vi "Kalp Atış Hızı Monitörü.vi"() -> ()   [LabVIEW 2017]
uses:
  <vilib>/LabVIEW Interface for Arduino/Type Defs/Digital Pin.ctl
  <vilib>/LabVIEW Interface for Arduino/Type Defs/Pin Mode.ctl
  <vilib>/LabVIEW Interface for Arduino/LabVIEW Interface for Arduino.lvlib
  <vilib>/ptbypt/NI_PtbyPt.lvlib
panel:
  out "Waveform Chart":u8(graph)
  out "Kalp Atımı":bool
  out "Kalp Atış Sayısı":i32
  in  "Çıkış":bool
  in  "Digital Pin":T1
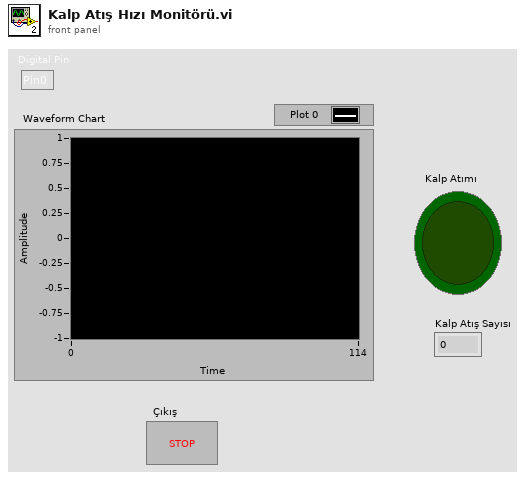
[diagram p1: front panel]
types:
  T1 = typedef "LabVIEW Interface for Arduino.lvlib/Digital Pin.ctl" = enum8{"Pin0", "Pin1", "Pin2", "Pin3", "Pin4", "Pin5", "Pin6", "Pin7", "Pin8", "Pin9", "Pin10", "Pin11", "Pin12", "Pin13"}
  T2 = typedef "LabVIEW Interface for Arduino.lvlib/Arduino Resource.ctl" = cluster{"VISA resource":refnum<visa-resource-name>, "Board Type":T3, "Connection Type":enum8{"USB / Serial"}, "Bytes Per Packet (15)":u8}
  T3 = typedef "LabVIEW Interface for Arduino.lvlib/Board Type.ctl" = enum16{"Uno", "Dimuelanove w/Atmega 328", "Mega 2560"}
  T4 = typedef "LabVIEW Interface for Arduino.lvlib/Pin Mode.ctl" = enum8{"Input", "Output"}
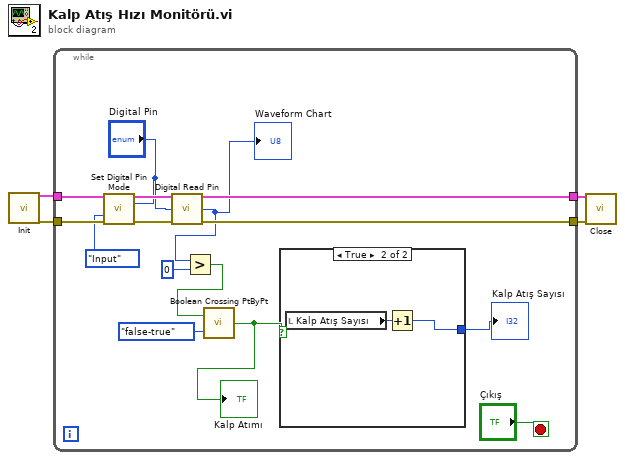
[diagram p0: block diagram]
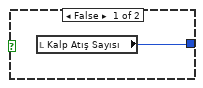
[diagram p2: hidden frame]
diagram:
  n1 = call <vilib>:"Init.vi"() -> ("Arduino Resource"=w2:T2, "error out"=w1:errorcluster)  [unwired: 18 in]
  n2 = while {
    tunnel: w2 -> [w15]
    tunnel: [w17] -> w4
    tunnel: w1 -> [w14]
    tunnel: [w16] -> w3
    stop <- "Çıkış" stop-if-true
    n3 = call <vilib>:"Set Digital Pin Mode.vi"("Arduino Resource"=w15, "Digital I/O Pin"="Digital Pin", "Pin Mode (Input)"=Pin_Mode."Input", "error in"=w14) -> ("Arduino Resource"=w19:T2, "error out"=w18:errorcluster)  [unwired: 10 in]
    n4 = call <vilib>:"Digital Read Pin.vi"("Arduino Resource"=w19, "Digital I/O Pin (0)"="Digital Pin", "error in"=w18) -> ("Arduino Resource"=w17:T2, "Value"=w5:u8, "error out"=w16:errorcluster)  [unwired: 10 in]
    "Waveform Chart" <- w5
    n5 = Greater?(x=w5, y=u8 0) -> (0:w10:bool)
    n6 = call <vilib>:"Boolean Crossing PtByPt.vi"("direction"=enum16{"either", "false-true", "true-false"}."false-true", "input"=w10) -> ("crossing"=w6:bool)  [unwired: 1 in]
    "Kalp Atımı" <- w6
    n7 = case shown="True" w6 {
      tunnel: [w20 w22] -> w7
      frame False {
        n8 = local read "Kalp Atış Sayısı"() -> (w20:i32)
      }
      frame True {
        n9 = local read "Kalp Atış Sayısı"() -> (w21:i32)
        n10 = Increment(x=w21) -> (x+1=w22:i32)
      }
    }
    "Kalp Atış Sayısı" <- w7
  }
  n11 = call <vilib>:"Close.vi"("Arduino Resource"=w4, "error in"=w3) -> ()  [unwired: 13 in, 1 out]
